vi "POS.vi"(8 "error in (no error)":errorcluster, 11 "VI Folder Path":path) -> (0 "error out":errorcluster, 2 "Balls":T1, 3 "Text":string)   [LabVIEW 2023]
panel:
  in  "Cluster":T2
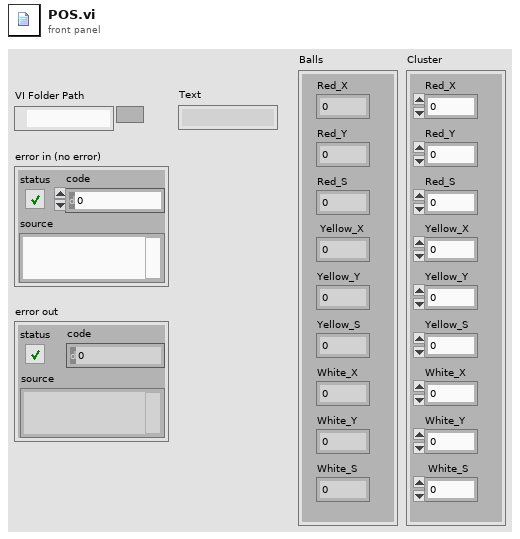
[diagram p1: front panel]
types:
  T1 = cluster{"Red_X":i32, "Red_Y":i32, "Red_S":i32, " Yellow_X":i32, "Yellow_Y":i32, "Yellow_S":i32, "White_X":i32, "White_Y":i32, "White_S":i32}
  T2 = cluster{"Red_X":i32, "Red_Y":i32, "Red_S":i32, "Yellow_X":i32, "Yellow_Y":i32, "Yellow_S":i32, "White_X":i32, "White_Y":i32, " White_S":i32}
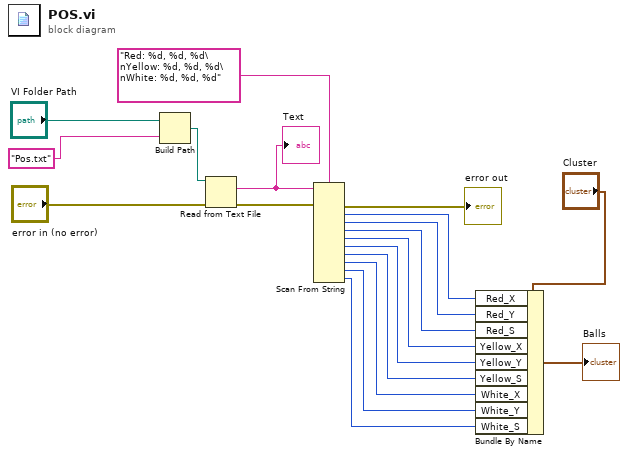
[diagram p0: block diagram]
diagram:
  n1 = Build Path(base path="VI Folder Path", name or relative path="Pos.txt") -> (appended path=w17:path)
  n2 = Read from Text File(file (use dialog)=w17, error in="error in (no error)") -> (text=w14:string, error out=w1:errorcluster)  [unwired: 2 in, 2 out]
  "Text" <- w14
  n3 = Scan From String(format string="Red: %d, %d, %d\nYellow: %d, %d, %d\nWhite: %d, %d, %d", input string=w14, error in=w1) -> (error out=→"error out":errorcluster, output 1=w12:i32, output 2=w10:i32, output 3=w9:i32, output 4=w8:i32, output 5=w7:i32, output 6=w6:i32, output 7=w5:i32, output 8=w4:i32, output 9=w3:i32)  [unwired: 10 in, 2 out]
  n4 = Bundle By Name(cluster="Cluster", "Red_X"=w12, "Red_Y"=w10, "Red_S"=w9, "Yellow_X"=w8, "Yellow_Y"=w7, "Yellow_S"=w6, "White_X"=w5, "White_Y"=w4, "White_S"=w3) -> (→"Balls":T2)
